vi "全局 反控命令枚举.vi"() -> ()   [LabVIEW 2016]
panel:
  in  "反控命令枚举":enum16{"返回请求应答", "返回执行结果"}(ring)
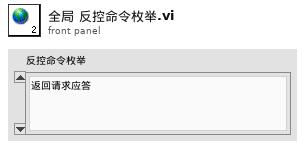
[diagram p1: front panel]
diagram:
